vi "xToString.vi"   [LabVIEW 2011]
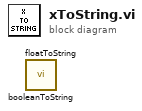
[diagram p0: block diagram]
diagram:
  n1 = call "booleanToString.vi"() -> ()  [unwired: 11 in, 1 out]
  n2 = call "floatToString.vi"() -> ()  [unwired: 11 in, 1 out]
